vi "Drive Get.vi"(1 "Change Gear?":bool, 2 "Left Y Axis":dbl, 3 "Axis Y Right":dbl, 4 "Axis X Right":dbl) -> ()   [LabVIEW 2012]
uses:
  Or David (Drive Global Data).vi
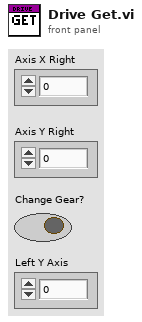
[diagram p1: front panel]
types:
  T1 = typedef "WPI_SolenoidValue.ctl" = enum16{"Off", "On", "Forward", "Reverse"}
  T2 = cluster{"Shifter?":bool, "Axisses":dbl[], "Shifter Value":T1}
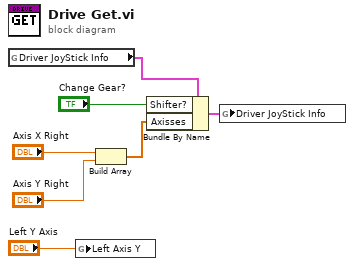
[diagram p0: block diagram]
diagram:
  n1 = global read "Or David (Drive Global Data).vi" "Driver JoyStick Info"() -> (w7:T2)
  n2 = global write "Or David (Drive Global Data).vi" "Left Axis Y"("Left Y Axis") -> ()
  n3 = Build Array("Axis X Right", "Axis Y Right") -> (w6:dbl[])
  n4 = Bundle By Name(cluster=w7, "Shifter?"="Change Gear?", "Axisses"=w6) -> (w4:T2)
  n5 = global write "Or David (Drive Global Data).vi" "Driver JoyStick Info"(w4) -> ()
